vi "IMAQdx_grab_att - Kopie (2).vi"() -> ()   [LabVIEW 2015]
doc: "The Grab VI acquires images continuously and displays the images in an image control using low-level acquisition VIs. A grab is appropriate for high-speed applications in which you need to process only one image at a time."
uses:
  <vilib>/userdefined/High Color/IMAQdx.ctl
  <vilib>/vision/driver/IMAQdx.llb/IMAQdx Attribute Type.ctl
  <vilib>/vision/driver/IMAQdx.llb/IMAQdx Acquisition Mode.ctl
  <vilib>/vision/driver/IMAQdx.llb/IMAQdx Buffer Number Mode.ctl
  <vilib>/vision/driver/NI_Vision_Acquisition_Software.lvlib
  <resource>/objmgr/imaqdx.rc
  <vilib>/vision/NI_Vision_Development_Module.lvlib
panel:
  in  "Exposure::Mode 3":u32(ring)=2 caption="Exposure::Mode" items=["Auto"=1, "Manual"=2]
  in  "stop":bool
  out "Exposure::Mode 2":u32(ring)=2 caption="Exposure::Mode" items=["Auto"=1, "Manual"=2]
  in  "String":string="um"
  out "output cluster":cluster{sgl, sgl}
  out "Last Mouse Position:All Elements":cluster{"X":i32, "Y":i32}
  in  "Gain::Value":i64 min=0 max=1728 step=1
  in  "Gain::Mode":u32(ring)=2 items=["Auto"=1, "Manual"=2]
  in  "Exposure::Value":dbl=0.0625 min=0.0 max=0.125
  in  "Exposure::Mode":u32(ring)=2 items=["Auto"=1, "Manual"=2]
  in  "Pixel Distances":T1={"X Step"=5.2, "Y Step"=5.2, "Unit"=enum."Micrometer"} {"Y Step" format="%.2f"; "X Step" format="%.2f"}
  out "Image Pixels (U8)":u8[][](array[numeric])
  out "error out":errorcluster
  out "Luminance Plane":T3(plugin-control)
  out "MinDBL":dbl
  out "MaxDBL":dbl
  out "Units":string
  out "GetExpVal":dbl
  out "Attribute Information Array":T5(array[cluster])
  out "IMAQdx Session":T6
  in  "Camera Name":refnum<k21>="cam0" caption="IMAQdx Session"
  out "Buffer Number":u32
  out "Image":T3(plugin-control)
  out "Frame Rate":dbl(knob) scale=0.0..20.0
  in  "Stop":bool
  # "Overview: Demonstrates how to acquire continuous images from a camera using low level acquisition functions.\nRequirements: Vision Acquisition Software\nInstructions:\n1. Select the Camera Name\n2. Run the VI"
  # "x /µm"
  # "y /µm"
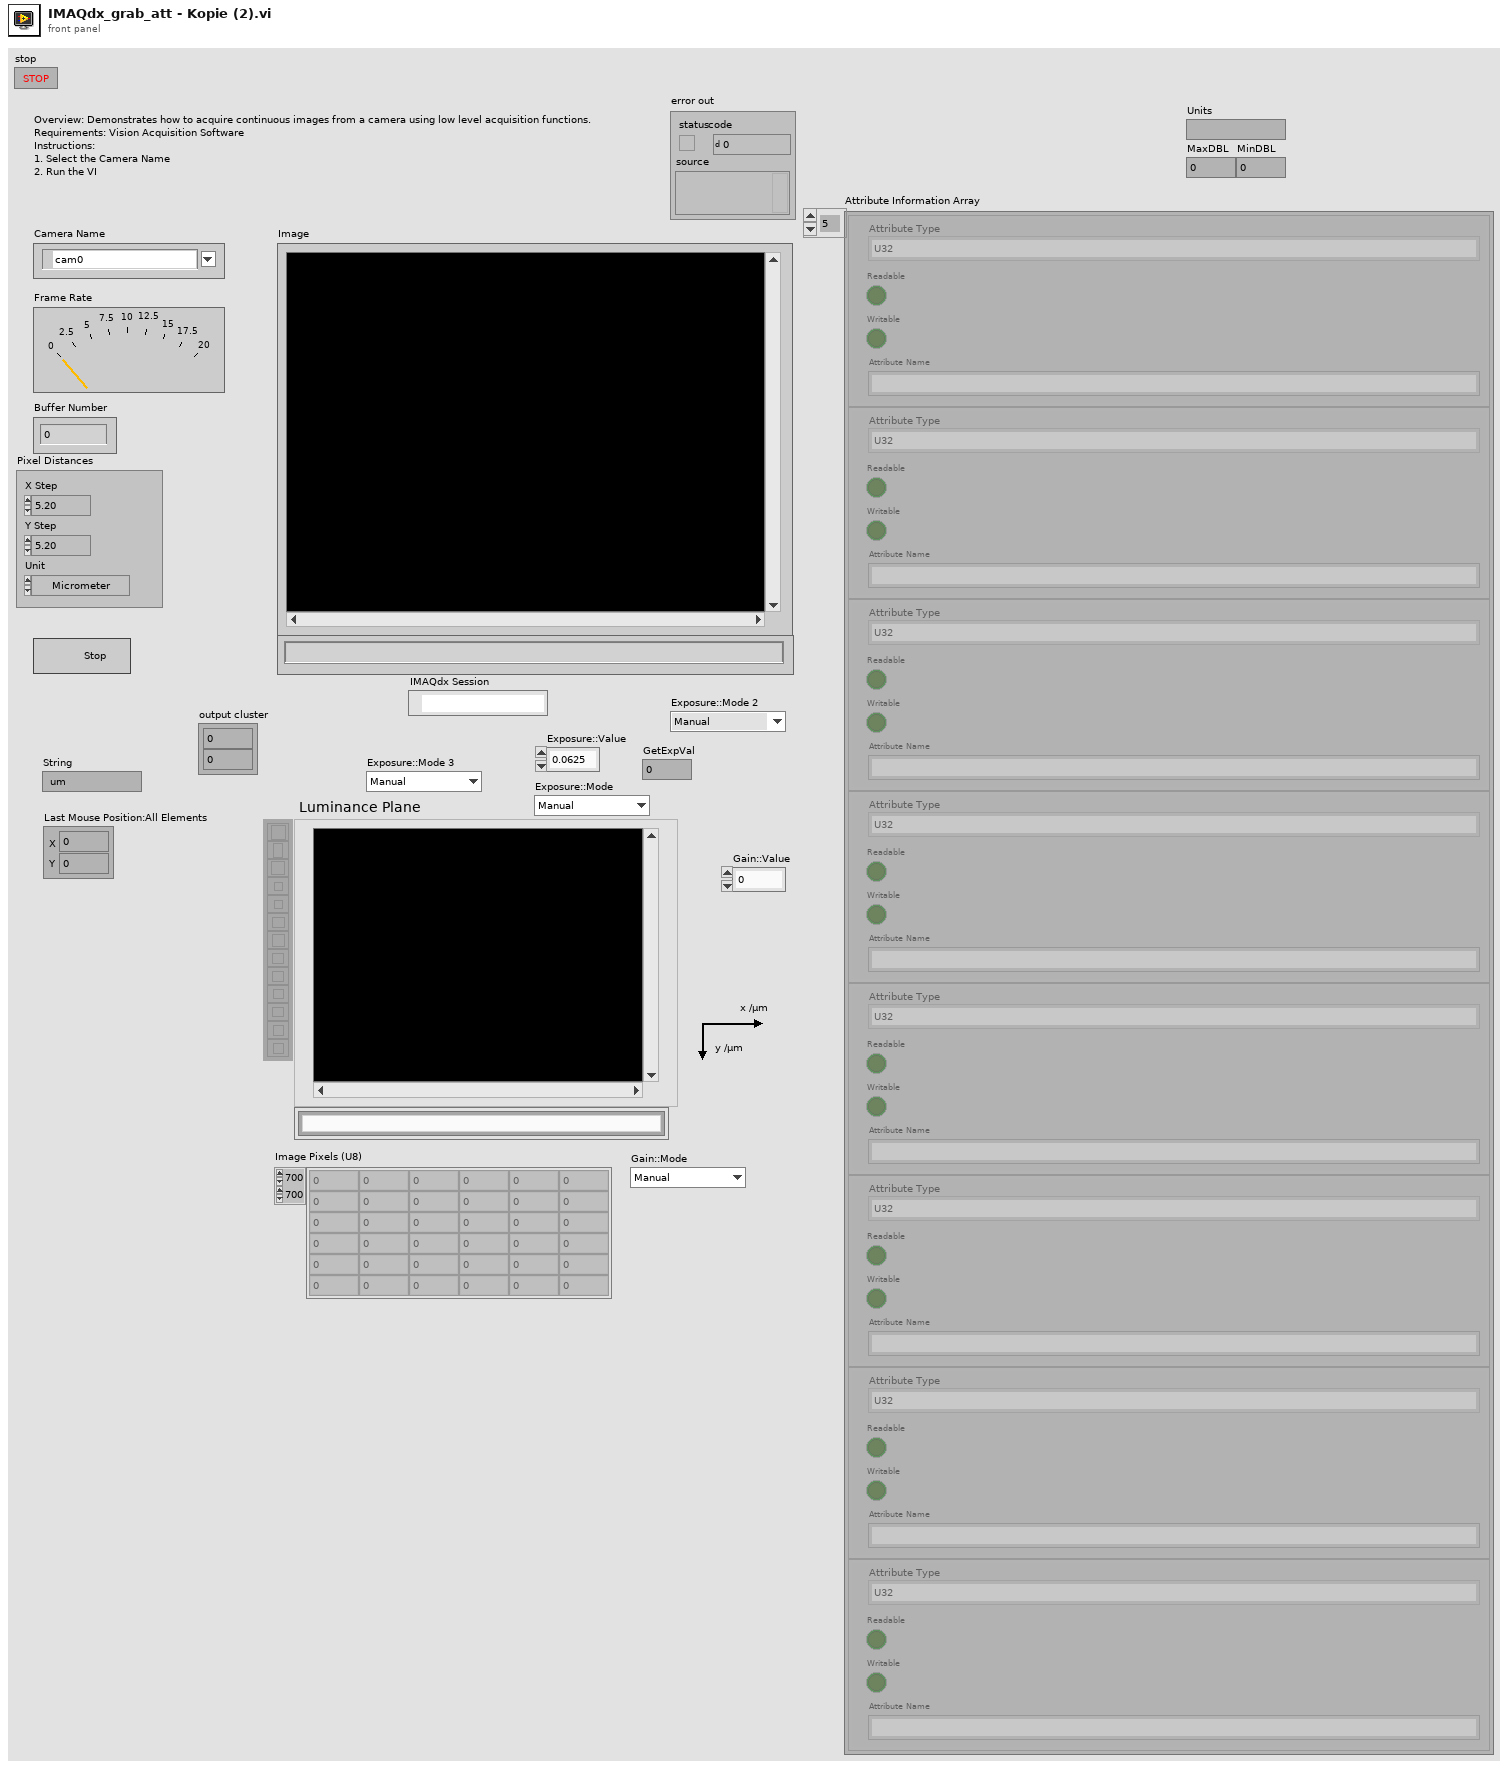
[diagram p1: front panel]
types:
  T1 = typedef "Simple Grid Descriptor" = cluster{"X Step":sgl, "Y Step":sgl, "Unit":T2}
  T2 = typedef "Image Unit" = enum32{"Undefined", "Angström", "Micrometer", "Millimeter", "Centimeter", "Meter", "Kilometer", "Microinch", "Inch", "Feet", "Nautical miles", "Standard miles", "Steps"}
  T3 = typedef "IMAQ Image.ctl" = refnum<image>
  T4 = typedef "NI_Vision_Acquisition_Software.lvlib/IMAQdx Attribute Type.ctl" = enum32{"U32", "I64", "DBL", "String", "Enum", "Bool", "Command"}
  T5 = cluster{"Attribute Type":T4, "Readable":bool, "Writable":bool, "Attribute Name":string}[]
  T6 = typedef "IMAQdx.ctl" = refnum<k21>
  T7 = typedef "Image Type" = u32
  T8 = typedef "NI_Vision_Acquisition_Software.lvlib/IMAQdx Acquisition Mode.ctl" = enum32{"One Shot", "Continuous"}
  T9 = typedef "NI_Vision_Acquisition_Software.lvlib/IMAQdx Buffer Number Mode.ctl" = enum32{"Next", "Last", "Buffer Number", "Every", "Last New"}
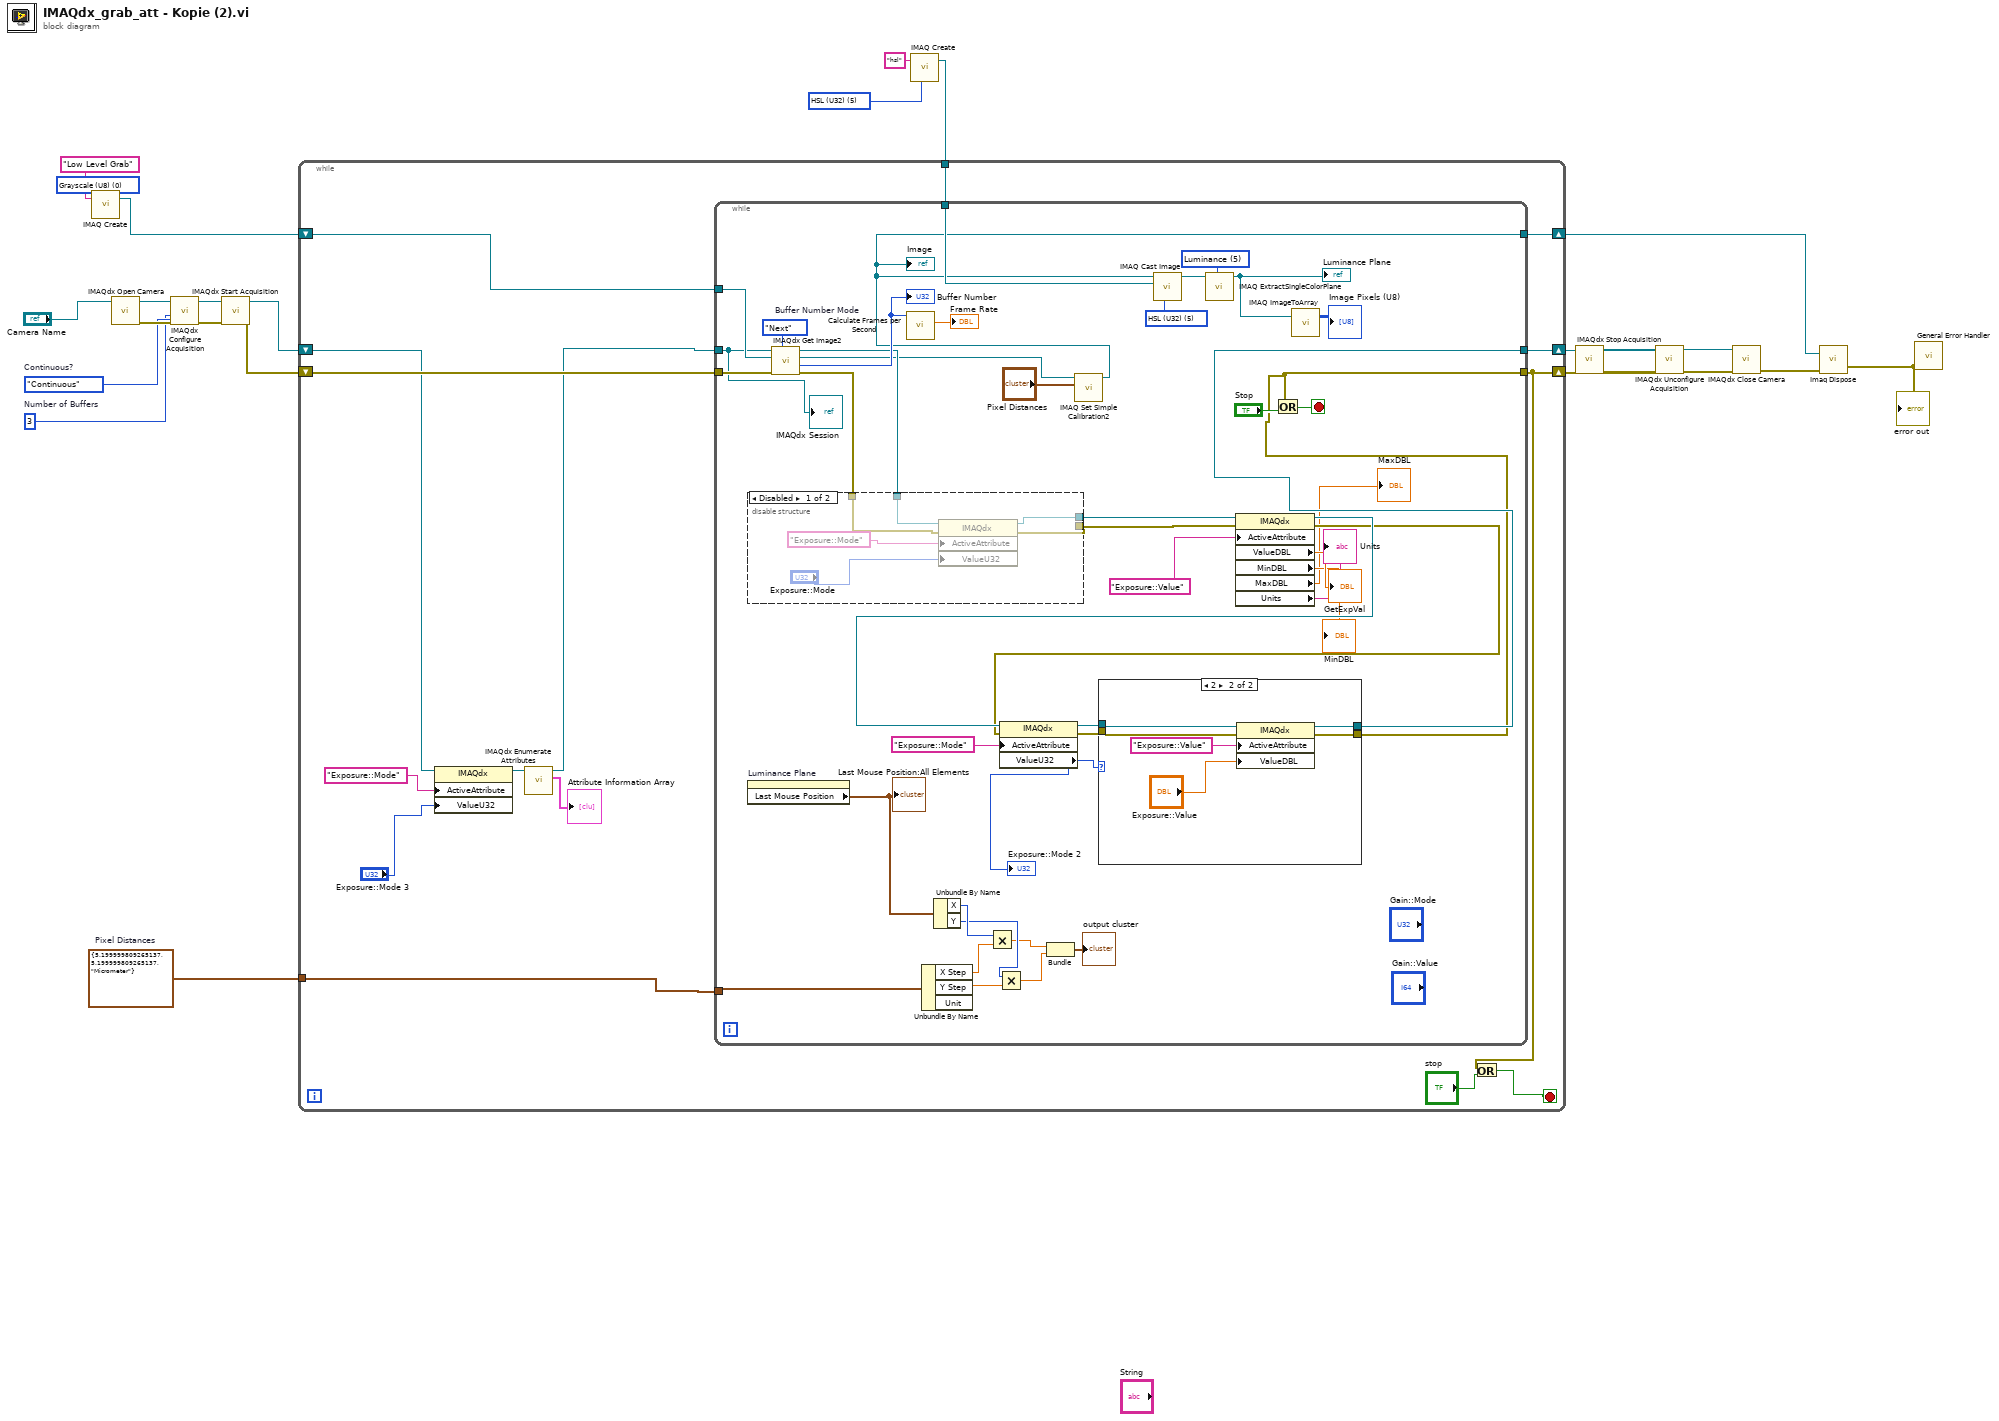
[diagram p0: block diagram]
diagram:
  w1 = T1 {"X Step"=5.2, "Y Step"=5.2, "Unit"=enum."Micrometer"}  # Pixel Distances
  w11 = T7 5 items=["Grayscale (U8)", "Grayscale (I16)", "Grayscale (SGL)", "Complex (CSG)", "RGB (U32)", "HSL (U32)", "RGB (U64)"] ("Image Type")
  w13 = T7 0 items=["Grayscale (U8)", "Grayscale (I16)", "Grayscale (SGL)", "Complex (CSG)", "RGB (U32)", "HSL (U32)", "RGB (U64)", "Grayscale (U16)"] ("Image Type")
  w21 = u32 3  # Number of Buffers
  w22 = IMAQdx_Acquisition_Mode."Continuous"  # Continuous?
  n1 = call "IMAQ Create"("Image Name"="Low Level Grab", "Image Type"=w13) -> ("New Image"=w25:T3)  [unwired: 2 in, 2 out]
  n2 = call <vilib>:"IMAQdx Open Camera.vi"("Session In"="Camera Name") -> ("error out"=w23:errorcluster, "Session Out"=w14:T6)  [unwired: 2 in, 7 out]
  n3 = call <vilib>:"IMAQdx Configure Acquisition.vi"("error in"=w23, "Number of Buffers"=w21, "Continuous?"=w22, "Session In"=w14) -> ("error out"=w9:errorcluster, "Session Out"=w3:T6)  [unwired: 6 out]
  n4 = call <vilib>:"IMAQdx Start Acquisition.vi"("error in"=w9, "Session In"=w3) -> ("error out"=w8:errorcluster, "Session Out"=w2:T6)  [unwired: 8 out]
  n5 = call "IMAQ Create"("Image Name"="hsl", "Image Type"=w11) -> ("New Image"=w10:T3)  [unwired: 3 in, 1 out]
  n6 = while {
    tunnel: w10 -> [w38]
    shift-right: [w39] -> w15
    shift-left: w25 -> [w40]
    shift-right: [w28] -> w7
    shift-left: w8 -> [w37]
    shift-right: [w36] -> w6
    shift-left: w2 -> [w32]
    tunnel: w1 -> [w27]
    stop <- w29 stop-if-true
    n7 = property class="IMAQdx"(reference=w32, "ActiveAttribute"="Exposure::Mode", "ValueU32"="Exposure::Mode 3") -> (reference out=w33:T6)  [unwired: 1 in, 1 out]
    n8 = call <vilib>:"IMAQdx Enumerate Attributes.vi"("Session In"=w33) -> ("Attribute Information Array"=→"Attribute Information Array":T5, "Session Out"=w31:T6)  [unwired: 8 in, 1 out]
    n9 = while {
      tunnel: [w70] -> w36
      tunnel: w37 -> [w82]
      tunnel: w31 -> [w76]
      tunnel: [w69] -> w28
      tunnel: w40 -> [w81]
      tunnel: [w54] -> w39
      tunnel: w38 -> [w57]
      tunnel: w27 -> [w51]
      stop <- w83 stop-if-true
      w59 = 5 items=["Red", "Green", "Blue", "Hue", "Saturation", "Luminance", "Value", "Intensity"] ("Color Plane")
      w60 = T7 5 items=["Grayscale (U8)", "Grayscale (I16)", "Grayscale (SGL)", "Complex (CSG)", "RGB (U32)", "HSL (U32)", "RGB (U64)"] ("Image Type")
      w79 = IMAQdx_Buffer_Number_Mode."Next"  # Buffer Number Mode
      n10 = property on="Luminance Plane" class="ImageControl"() -> ("Last Mouse Position"=w50:cluster{"X":i32, "Y":i32})  [unwired: 2 in, 2 out]
      "Last Mouse Position:All Elements" <- w50
      n11 = call <vilib>:"IMAQdx Get Image2.vi"("Buffer Number Mode (Next)"=w79, "error in"=w82, "Image In"=w81, "Session In"=w76) -> ("error out"=w72:errorcluster, "Buffer Number Out"=w78:u32, "Image Out"=w53:T3, "Session Out"=w71:T6)  [unwired: 4 in]
      "Buffer Number" <- w78
      n12 = disable-structure shown="Disabled" {
        disable-tunnel: [w88 w91] -> w74
        disable-tunnel: [w87 w90] -> w73
        disable-tunnel: w72 -> [w86 w90]
        disable-tunnel: w71 -> [w85 w91]
        frame Disabled {
          n13 = property class="IMAQdx"(reference=w85, error in=w86, "ActiveAttribute"="Exposure::Mode", "ValueU32"="Exposure::Mode") -> (reference out=w88:T6, error out=w87:errorcluster)
        }
        frame Enabled {
        }
      }
      n14 = call <vilib>:"Calculate Frames per Second.vi"("Buffer Number"=w78) -> ("Processed Frames/s"=→"Frame Rate":dbl)  [unwired: 8 in, 2 out]
      n15 = Unbundle By Name(w51) -> ("X Step"=w48:sgl, "Y Step"=w46:sgl)  [unwired: 1 out]
      n16 = Unbundle By Name(w50) -> ("X"=w49:i32, "Y"=w47:i32)
      n17 = Multiply(x=w49, y=w48) -> (x*y=w44:sgl)
      n18 = Multiply(x=w47, y=w46) -> (x*y=w45:sgl)
      n19 = Bundle(w44, w45) -> (→"output cluster":cluster{sgl, sgl})  [unwired: 1 in]
      n20 = call "IMAQ Set Simple Calibration2"("Pixel Distances"="Pixel Distances", "Image"=w53) -> ("Calibration Template Image"=w54:T3)  [unwired: 8 in, 1 out]
      "Image" <- w54
      n21 = call "IMAQ Cast Image"("Image Type"=w60, "Image Dst"=w57, "Image Src"=w54) -> ("Image Dst Out"=w58:T3)  [unwired: 7 in, 1 out]
      n22 = call "IMAQ ExtractSingleColorPlane"("Color Plane"=w59, "Image Src"=w58) -> ("Image Dst Out"=w52:T3)  [unwired: 8 in, 1 out]
      "Luminance Plane" <- w52
      n23 = property class="IMAQdx"(reference=w74, error in=w73, "ActiveAttribute"="Exposure::Value") -> (reference out=w66:T6, error out=w65:errorcluster, "ValueDBL"=→"GetExpVal":dbl, "MinDBL"=→"MinDBL":dbl, "MaxDBL"=→"MaxDBL":dbl, "Units"=→"Units":string)
      n24 = property class="IMAQdx"(reference=w66, error in=w65, "ActiveAttribute"="Exposure::Mode") -> (reference out=w64:T6, error out=w63:errorcluster, "ValueU32"=w41:u32)
      "Exposure::Mode 2" <- w41
      n25 = case shown="2" w41 {
        tunnel: w64 -> [w93 w98]
        tunnel: w63 -> [w92 w97]
        tunnel: [w93 w96] -> w70
        tunnel: [w92 w95] -> w69
        frame 1, Default {
        }
        frame 2 {
          n26 = property class="IMAQdx"(reference=w98, error in=w97, "ActiveAttribute"="Exposure::Value", "ValueDBL"="Exposure::Value") -> (reference out=w96:T6, error out=w95:errorcluster)
        }
      }
      n27 = Or(x=w69, y="Stop") -> (x .or. y?=w83:bool)
      n28 = call "IMAQ ImageToArray"("Image"=w52) -> ("Image Pixels (U8)"=→"Image Pixels (U8)":u8[][])  [unwired: 3 in, 4 out]
      "IMAQdx Session" <- w76
    }
    n29 = Or(x=w28, y="stop") -> (x .or. y?=w29:bool)
  }
  n30 = call <vilib>:"IMAQdx Stop Acquisition.vi"("error in"=w7, "Session In"=w6) -> ("error out"=w4:errorcluster, "Session Out"=w5:T6)  [unwired: 8 out]
  n31 = call <vilib>:"IMAQdx Unconfigure Acquisition.vi"("error in"=w4, "Session In"=w5) -> ("error out"=w20:errorcluster, "Session Out"=w19:T6)  [unwired: 8 out]
  n32 = call <vilib>:"IMAQdx Close Camera.vi"("error in"=w20, "Session In"=w19) -> ("error out"=w18:errorcluster)  [unwired: 9 out]
  n33 = call "Imaq Dispose"("Image"=w15, "error in (no error)"=w18) -> ("error out"=w17:errorcluster)  [unwired: 4 in]
  "error out" <- w17
  n34 = call <vilib>:"General Error Handler.vi"("error in (no error)"=w17) -> ()  [unwired: 2 in, 13 out]
